vi "Get Frames and Signals from Clusters.vi"(0 "XNET Clusters":refnum<k21>[](array[refnum]), 11 "error in":errorcluster) -> (2 "Number of Clusters":i32, 3 "Number of Frames":i32[](array[numeric]), 4 "Cluster Names":string[](array[string]), 6 "Frame Names":string[][](array[string]), 8 "Signal Names":string[][][](array[string]), 14 "Number of Signals":i32[][](array[numeric]), 15 "error out":errorcluster)   [LabVIEW 2015]
uses:
  <resource>/objmgr/xnet.rc
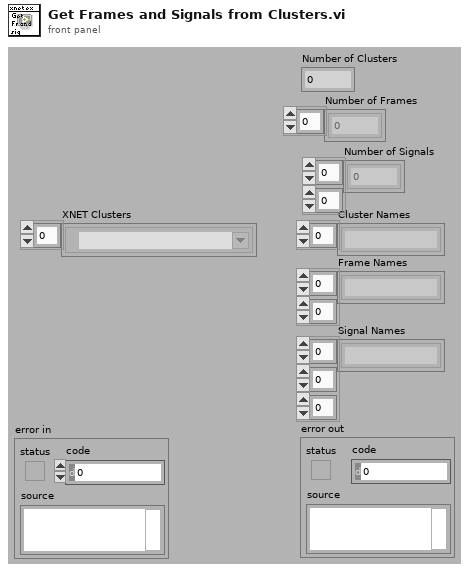
[diagram p1: front panel]
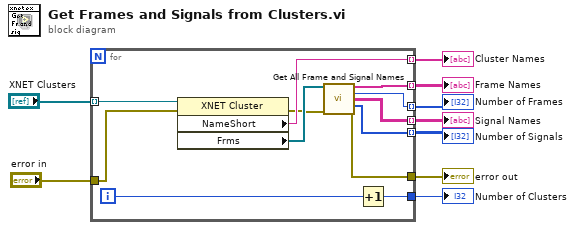
[diagram p0: block diagram]
diagram:
  n1 = for {
    tunnel: "XNET Clusters" -> [w11] mode=indexing
    tunnel: "error in" -> [w10]
    tunnel: [w18] -> w5 mode=indexing
    tunnel: [w21] -> w9 mode=indexing
    tunnel: [w17] -> w6
    tunnel: [w16] -> w4 mode=indexing
    tunnel: [w15] -> w3 mode=indexing
    tunnel: [w14] -> w2 mode=indexing
    tunnel: [w13] -> w1
    i -> [w12]
    n2 = property class="XNET Cluster"(reference=w11, error in=w10) -> (error out=w19:errorcluster, "NameShort"=w21:string, "Frms"=w20:refnum<k21>[])  [unwired: 1 out]
    n3 = call "Get All Frame and Signal Names.vi"("XNET Frames"=w20, "error in"=w19) -> ("Frame Names"=w18:string[], "Number of Frames"=w15:i32, "Signal Names"=w16:string[][], "Number of Signals"=w14:i32[], "error out"=w17:errorcluster)  [unwired: 9 in]
    n4 = Increment(x=w12) -> (x+1=w13:i32)
  }
  "Cluster Names" <- w9
  "Frame Names" <- w5
  "Signal Names" <- w4
  "error out" <- w6
  "Number of Clusters" <- w1
  "Number of Frames" <- w3
  "Number of Signals" <- w2
